vi "Caps_GUI.vi"(10 "stop 2":refnum<vi>, 11 "GUI_cluster":T1={"Sub Panel"=refnum, "GUIdevice"="Bella_LP_Mode", "CtlRef"=refnum, "user event out"=refnum}) -> ()   [LabVIEW 2011]
uses:
  GUI_Template/GUI_master/tcp_new_data_event.ctl
  GUI_Template/GUI_master/tcp new data cluster.ctl
  Controls/GUI_cluster.ctl
  Controls/eventtypdef.ctl
panel:
  out "GUIdevice 7":string="StagingInterlock"
  in  "installed.cap2::7":bool caption="CAP2 installed"
  in  "installed.cap1::7":bool caption="CAP1 installed"
  out "read voltage 2":dbl=-0.022297334844 caption="read \nvoltage" min=0.0 max=0.0
  out "read voltage":dbl=0.036783739484999994 caption="read \nvoltage" min=0.0 max=0.0
  out "GUIdevice 6":string="StagingAnalysisSlow"
  out "GUIdevice 5":string="StagingLowPressure2"
  out "GUIdevice 4":string="StagingLowPressure1"
  out "GUIdevice 3":string="StagingNISwitch"
  out "GUIdevice 2":string="StagingDischargePower"
  out "timing (ns) 2":dbl
  in  "timing (ns)":dbl
  out "pressureCap1::6":dbl=74.657900037871 caption="pressure read" min=0.0 max=10.0
  out "pressureCap2::6":dbl=77.24427975638 caption="pressure read" min=0.0 max=10.0
  in  "pressure::5":dbl=74.96 caption="pressure" min=0.0 max=200.0
  in  "pressure::4":dbl=75.28 caption="pressure" min=0.0 max=200.0
  in  "discharge2::3":bool caption="Trigger"
  in  "discharge1::3":bool caption="Trigger"
  out "AI_mean.Channel 3::2":dbl=0.012277955671 caption="read \nvoltage" min=0.0 max=0.0
  in  "voltage.hv 2::1":dbl=0.040871 caption="set \nvoltage" min=0.0 max=30.0
  out "AI_mean.Channel 0::2":dbl=-0.007397741276 caption="read \nvoltage" min=0.0 max=0.0
  in  "voltage.hv 1::1":dbl=-0.024775 caption="set \nvoltage" min=0.0 max=30.0
  out "tcp data event":T2
  out "GUIdevice 1":string="StagingDischargeHV"
  in  "stop":bool=TRUE
  # "CAP2"
  # "CAP1"
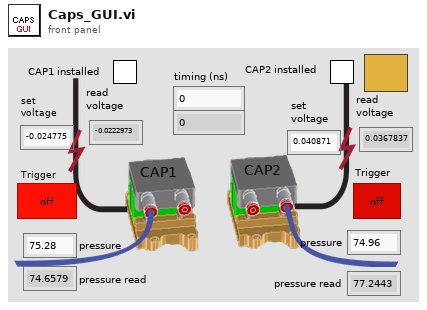
[diagram p1: front panel]
types:
  T1 = typedef "GUI_cluster.ctl" = cluster{"Sub Panel":refnum<vi>, "GUIdevice":string, "CtlRef":refnum<vi>, "user event out":refnum<user-event>}
  T2 = typedef "tcp_new_data_event.ctl" = refnum<user-event>
  T3 = typedef "eventtypdef.ctl" = cluster{"label":string, "Sub Panel":refnum<vi>, "CtlRef":refnum<vi>, "This VI":refnum<vi>}
  T4 = typedef "tcp new data cluster.ctl" = cluster{"EventEnum":enum16{"new data", "connection status update"}, "Device name":string}
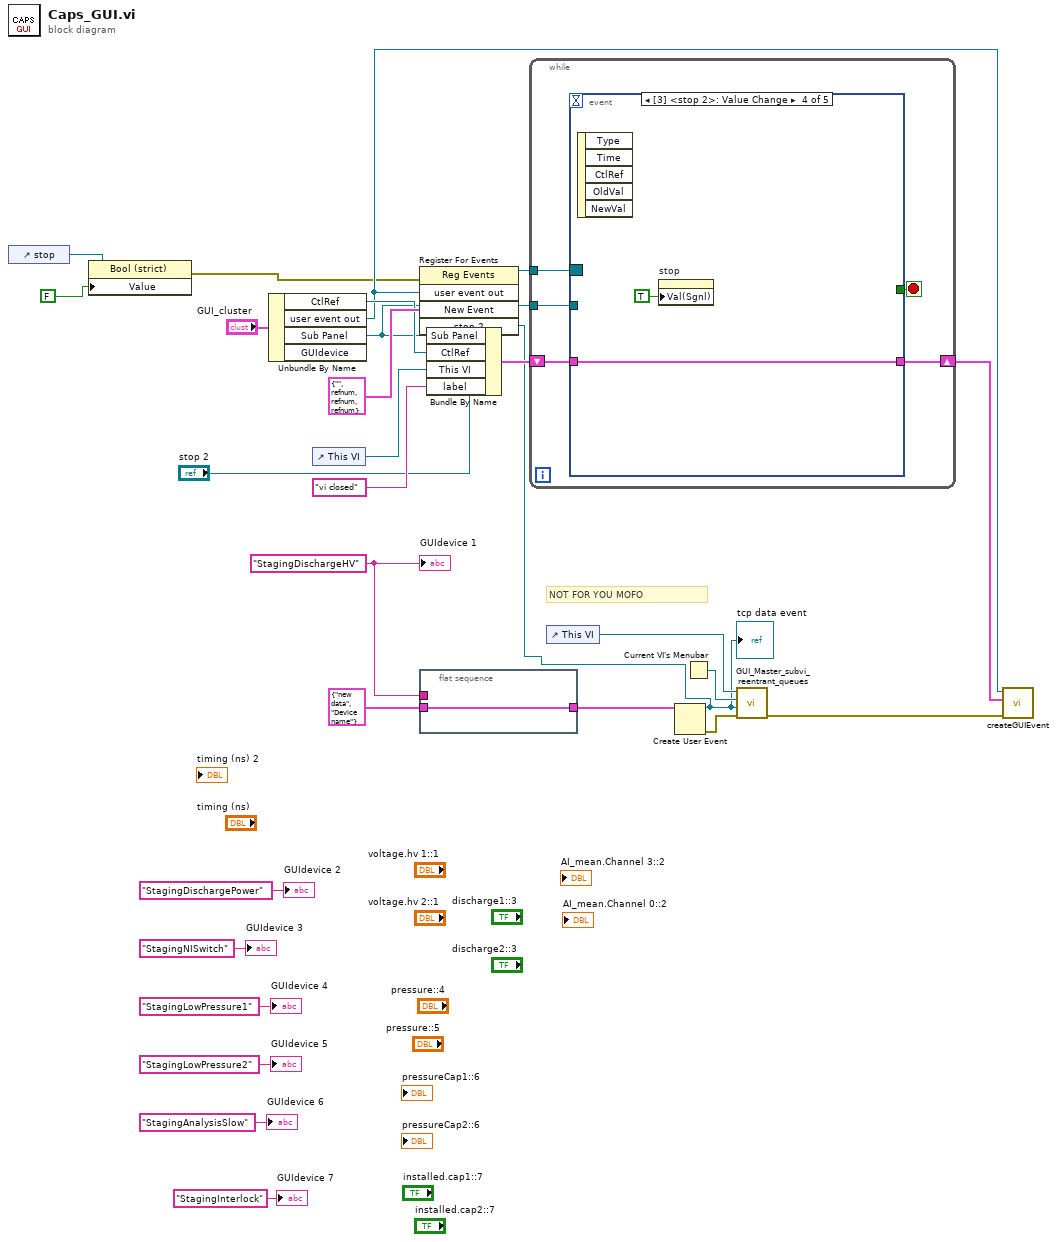
[diagram p0: block diagram]
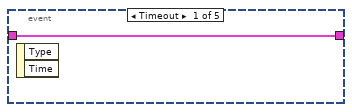
[diagram p2: hidden frame]
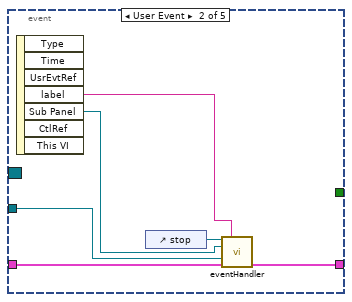
[diagram p3: hidden frame]
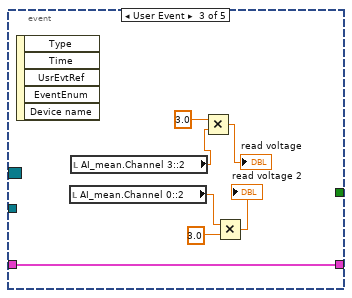
[diagram p4: hidden frame]
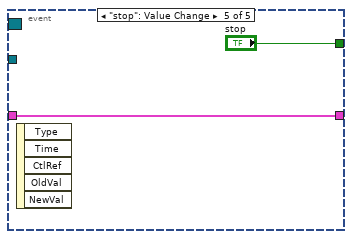
[diagram p5: hidden frame]
diagram:
  w19 = "StagingDischargeHV" ("GUIdevice 23")
  # "NOT FOR YOU MOFO"
  n1 = control-ref of="stop"() -> (w4:refnum<vi>)
  n2 = property class="Bool (strict)"(reference=w4, "Value"=FALSE) -> (error out=w2:errorcluster)  [unwired: 1 in, 1 out]
  n3 = Unbundle By Name("GUI_cluster") -> ("CtlRef"=w21:refnum<vi>, "user event out"=w8:refnum<user-event>, "Sub Panel"=w11:refnum<vi>)  [unwired: 1 out]
  n4 = control-ref of="This VI"() -> (w20:refnum<vi>)
  n5 = flat-sequence {
    tunnel: T4 {"EventEnum"=enum."new data", "Device name"="Device name"} ("New Event") -> [w29]
    tunnel: [w29] -> w22
    tunnel: w19 -> [_]
    frame #0 {
    }
  }
  n6 = Bundle By Name(cluster=T3 {"label"="", "Sub Panel"=refnum, "CtlRef"=refnum, "This VI"=refnum} ("event data"), "Sub Panel"=w11, "CtlRef"=w21, "This VI"=w20, "label"="vi closed") -> (w10:T3)
  n7 = control-ref of="This VI"() -> (w28:refnum<vi>)
  n8 = Create User Event(user event datatype=w22) -> (user event=w6:refnum<user-event>, error out=w26:errorcluster)  [unwired: 1 in]
  "tcp data event" <- w6
  n9 = register-events(error in=w2, w8, w6, "stop 2") -> (reference out=w13:refnum<event-registration>)  [unwired: 1 in, 1 out]
  n10 = while {
    tunnel: w13 -> [w34]
    tunnel: w11 -> [w32]
    shift-right: [w30] -> w7
    shift-left: w10 -> [w31]
    stop <- w33 stop-if-true
    n11 = event shown="[3] <stop 2>: Value Change" {
      selector: w34 -> [_ _ _ _ _]
      dyn-events: _ -> [_ _ _ _ _]
      timeout: _ -> [_ _ _ _ _]
      tunnel: [_ _ _ _ "stop"] -> w33
      tunnel: w32 -> [_ w38 _ _ _]
      tunnel: w31 -> [w35 w37 w42 w50 w51]
      tunnel: [w35 w36 w42 w50 w51] -> w30
      event Timeout {
        n12 = event-data() -> ()  [unwired: 1 in, 2 out]
      }
      event User Event {
        n13 = event-data() -> ("label"=w40:string, "Sub Panel"=w39:refnum<vi>)  [unwired: 1 in, 5 out]
        n14 = control-ref of="stop"() -> (w41:refnum<vi>)
        n15 = call "eventHandler.vi"("Boolean in"=w41, "label"=w40, "Sub Panel 2"=w39, "Sub Panel"=w38, "event data in"=w37) -> ("event data out"=w36:T3)  [unwired: 10 in]
      }
      event User Event {
        n16 = event-data() -> ()  [unwired: 1 in, 5 out]
        n17 = local read "AI_mean.Channel 0::2"() -> (w45:dbl)
        n18 = local read "AI_mean.Channel 3::2"() -> (w48:dbl)
        n19 = Multiply(x=3.0, y=w48) -> (x*y=→"read voltage":dbl)
        n20 = Multiply(x=w45, y=3.0 ("x")) -> (x*y=→"read voltage 2":dbl)
      }
      event Value Change {
        n21 = event-data() -> ()  [unwired: 1 in, 5 out]
        n22 = property on="stop" class="Bool (strict)"("Val(Sgnl)"=TRUE ("Value (Signaling)")) -> ()  [unwired: 2 in, 2 out]
      }
      event "stop": Value Change {
        n23 = event-data() -> ()  [unwired: 1 in, 5 out]
      }
    }
  }
  n24 = Current VI's Menubar() -> (w27:refnum<k9>)
  n25 = call "GUI_Master_subvi_reentrant_queues.vi"("error in (no error)"=w26, "tcp data event"=w6, "Caller menu reference"=w27, "Caller VI ref"=w28) -> ("error out"=w9:errorcluster)  [unwired: 7 in]
  n26 = call "createGUIEvent.vi"("error in (no error)"=w9, "event data"=w7, "User Event in"=w8) -> ()  [unwired: 9 in]
  "GUIdevice 1" <- w19
  "GUIdevice 2" <- "StagingDischargePower" ("GUIdevice 23")
  "GUIdevice 3" <- "StagingNISwitch" ("GUIdevice 8")
  "GUIdevice 4" <- "StagingLowPressure1" ("GUIdevice 2")
  "GUIdevice 5" <- "StagingLowPressure2" ("GUIdevice 2")
  "GUIdevice 6" <- "StagingAnalysisSlow" ("GUIdevice 1")
  "GUIdevice 7" <- "StagingInterlock" ("GUIdevice 7")
